vi "Deps.vi"   [LabVIEW 2020, in "HTTP Server.lvlib" / "Server.lvclass"]
uses:
  Server.lvclass
  Processing/Processing.lvclass
  Session/Session.lvclass
  Values/Values.lvclass
  WebSocket Handler/WebSocket Handler.lvclass
  RequestTraceLog/RequestTraceLog.lvclass
  Authentication Provider/Authentication Provider.lvclass
  Password Encoder/Password Encoder.lvclass
  User Provider/User Provider.lvclass
  User/User.lvclass
  Complete Handler/Complete Handler.lvclass
  Connection Handler/Connection Handler.lvclass
  Controller Handler/Controller Handler.lvclass
  Exception Handler/Exception Handler.lvclass
  Request Handler/Request Handler.lvclass
  Response Handler/Response Handler.lvclass
  Route Handler/Route Handler.lvclass
  Controller/Controller.lvclass
  Handler/Handler.lvclass
  Service/Service.lvclass
  StandardFileServe/StandardFileServe.lvclass
  Caching Complete/Caching Complete.lvclass
  Caching Request/Caching Request.lvclass
  Caching Response/Caching Response.lvclass
  Caching/Caching.lvclass
  BasicPasswordEncoder/BasicPasswordEncoder.lvclass
  FormAuthentication/FormAuthentication.lvclass
  Security/Security.lvclass
  Authentication Handler/Authentication Handler.lvclass
  BadRequestException/BadRequestException.lvclass
  FileNotFoundException/FileNotFoundException.lvclass
  NoControllerException/NoControllerException.lvclass
  Request Session Handler/Request Session Handler.lvclass
  Session Cleanup Handler/Session Cleanup Handler.lvclass
  Session Response Handler/Session Response Handler.lvclass
  ControllerIndexedPathParams Handler/ControllerIndexedPathParams Handler.lvclass
  FileExistChecker/FileExistChecker.lvclass
  HTTPS Redirect Handler/HTTPS Redirect Handler.lvclass
  PathRegex Router/PathRegex Router.lvclass
  PathValidation/PathValidation.lvclass
  Process Async.vi
  Server.lvclass/Server.ctl
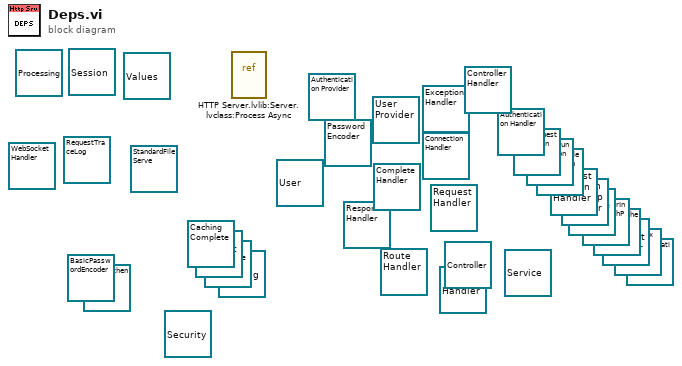
[diagram p0: block diagram]
diagram:
  (unwired) refnum<class "PathValidation.lvclass"> refnum ("HTTP Server:PathValidation.lvclass")
  (unwired) refnum<class "PathRegex Router.lvclass"> refnum ("HTTP Server:PathRegex Router.lvclass")
  (unwired) refnum<class "HTTPS Redirect Handler.lvclass"> refnum ("HTTP Server:HTTPS Redirect Handler.lvclass")
  (unwired) refnum<class "FileExistChecker.lvclass"> refnum ("HTTP Server:FileExistChecker.lvclass")
  (unwired) refnum<class "ControllerIndexedPathParams Handler.lvclass"> refnum ("HTTP Server:ControllerIndexedPathParams Handler.lvclass")
  (unwired) refnum<class "Session Response Handler.lvclass"> refnum ("HTTP Server:Session Response Handler.lvclass")
  (unwired) refnum<class "Session Cleanup Handler.lvclass"> refnum ("HTTP Server:Session Cleanup Handler.lvclass")
  (unwired) refnum<class "Request Session Handler.lvclass"> refnum ("HTTP Server:Request Session Handler.lvclass")
  (unwired) refnum<class "NoControllerException.lvclass"> refnum ("HTTP Server:NoControllerException.lvclass")
  (unwired) refnum<class "FileNotFoundException.lvclass"> refnum ("HTTP Server:FileNotFoundException.lvclass")
  (unwired) refnum<class "BadRequestException.lvclass"> refnum ("HTTP Server:BadRequestException.lvclass")
  (unwired) refnum<class "Authentication Handler.lvclass"> refnum ("HTTP Server:Authentication Handler.lvclass")
  (unwired) refnum<class "Security.lvclass"> refnum ("HTTP Server:Security.lvclass")
  (unwired) refnum<class "FormAuthentication.lvclass"> refnum ("HTTP Server:FormAuthentication.lvclass")
  (unwired) refnum<class "BasicPasswordEncoder.lvclass"> refnum ("HTTP Server:BasicPasswordEncoder.lvclass")
  (unwired) refnum<class "Caching.lvclass"> refnum ("HTTP Server:Caching.lvclass")
  (unwired) refnum<class "Caching Response.lvclass"> refnum ("HTTP Server:Caching Response.lvclass")
  (unwired) refnum<class "Caching Request.lvclass"> refnum ("HTTP Server:Caching Request.lvclass")
  (unwired) refnum<class "Caching Complete.lvclass"> refnum ("HTTP Server:Caching Complete.lvclass")
  (unwired) refnum<class "StandardFileServe.lvclass"> refnum ("HTTP Server:StandardFileServe.lvclass")
  (unwired) refnum<class "Service.lvclass"> refnum ("HTTP Server:Service.lvclass")
  (unwired) refnum<class "Handler.lvclass"> refnum ("HTTP Server:Handler.lvclass")
  (unwired) refnum<class "Controller.lvclass"> refnum ("HTTP Server:Controller.lvclass")
  (unwired) refnum<class "Route Handler.lvclass"> refnum ("HTTP Server:Route Handler.lvclass")
  (unwired) refnum<class "Response Handler.lvclass"> refnum ("HTTP Server:Response Handler.lvclass")
  (unwired) refnum<class "Request Handler.lvclass"> refnum ("HTTP Server:Request Handler.lvclass")
  (unwired) refnum<class "Exception Handler.lvclass"> refnum ("HTTP Server:Exception Handler.lvclass")
  (unwired) refnum<class "Controller Handler.lvclass"> refnum ("HTTP Server:Controller Handler.lvclass")
  (unwired) refnum<class "Connection Handler.lvclass"> refnum ("HTTP Server:Connection Handler.lvclass")
  (unwired) refnum<class "Complete Handler.lvclass"> refnum ("HTTP Server:Complete Handler.lvclass")
  (unwired) refnum<class "User.lvclass"> refnum ("HTTP Server:User.lvclass")
  (unwired) refnum<class "User Provider.lvclass"> refnum ("HTTP Server:User Provider.lvclass")
  (unwired) refnum<class "Password Encoder.lvclass"> refnum ("HTTP Server:Password Encoder.lvclass")
  (unwired) refnum<class "Authentication Provider.lvclass"> refnum ("HTTP Server:Authentication Provider.lvclass")
  (unwired) refnum<class "RequestTraceLog.lvclass"> refnum ("HTTP Server:RequestTraceLog.lvclass")
  (unwired) refnum<class "WebSocket Handler.lvclass"> refnum ("HTTP Server:WebSocket Handler.lvclass")
  (unwired) refnum<class "Values.lvclass"> refnum ("HTTP Server:Values.lvclass")
  (unwired) refnum<class "Session.lvclass"> refnum ("HTTP Server:Session.lvclass")
  (unwired) refnum<class "Processing.lvclass"> refnum ("HTTP Server:Processing")
  n1 = vi-ref "HTTP Server.lvlib:Server.lvclass:Process Async.vi"() -> ()  [unwired: 1 out]
